vi "Write tcsGuideCorrectionTime.vi"(8 "error in (no error)":errorcluster, 10 "tcsGuideCorrectionTime":timestamp, 11 "GuiderMeasuredError in":refnum<class "GuiderMeasuredError.lvclass">) -> (0 "error out":errorcluster, 3 "GuiderMeasuredError out":refnum<class "GuiderMeasuredError.lvclass">)   [LabVIEW 2022 SP3, in "TCSDataDefinitions.lvlib" / "TCSGuiderCommand.lvlib" / "GuiderMeasuredError.lvclass"]
uses:
  GuiderMeasuredError.lvclass
  GuiderMeasuredError.lvclass/GuiderMeasuredError.ctl
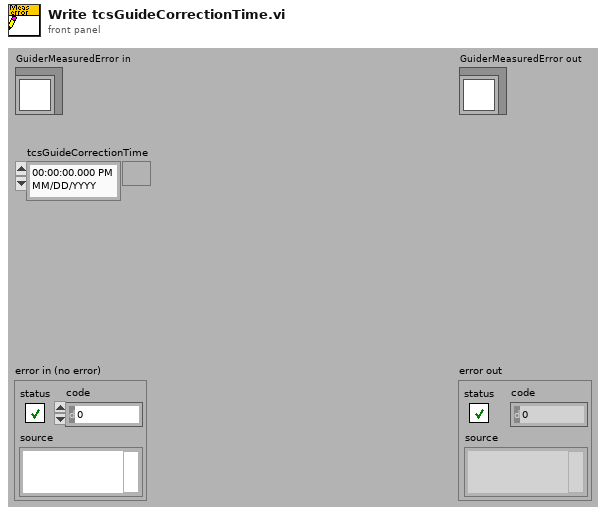
[diagram p1: front panel]
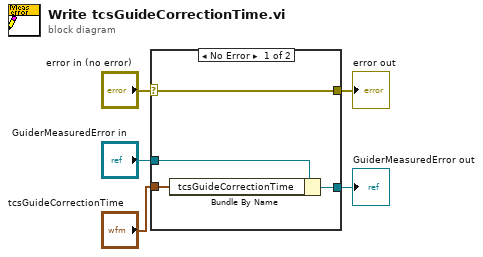
[diagram p0: block diagram]
diagram:
  n1 = case shown="No Error" "error in (no error)" {
    selector: "error in (no error)" -> [w9 w10]
    tunnel: [w9 w10] -> w4
    tunnel: [w7 w11] -> w2
    tunnel: "GuiderMeasuredError in" -> [w8 w11]
    tunnel: "tcsGuideCorrectionTime" -> [w6 _]
    frame No Error {
      n2 = Bundle By Name(cluster=w8, "tcsGuideCorrectionTime"=w6) -> (w7:refnum<class "GuiderMeasuredError.lvclass">)
    }
    frame Error {
    }
  }
  "error out" <- w4
  "GuiderMeasuredError out" <- w2
